vi "Custom Aggregation (Symm Comp).vi"(0 "symmetrical components":T2, 1 "reset? (F)":bool, 5 "aggregation settings":T1={"interval"=1, "interval unit"=enum."Runs", "synchronization of intervals"=enum."Not synchronized", "algorithm"=enum."Average"}, 9 "system info in":refnum<class "EP System Info.lvclass">, 11 "error in (no error)":errorcluster, 12 "data timestamp":timestamp) -> (4 "aggregated minimum value":T2, 6 "aggregated averaged/RMS value":T2, 8 "aggregated maximum value":T2, 10 "system info out":refnum<class "EP System Info.lvclass">, 13 "aggregated data valid?":bool, 14 "aggregated data timestamp":timestamp, 15 "error out":errorcluster)   [LabVIEW 2014, in "NI_EP_Power Quality.lvlib"]
doc: "Calculates the aggregated minimum, maximum, and averaged or RMS value of an input signal for a specified aggregation interval, according to Class S in IEC 61000-4-30:2008. There is no overlap between aggregation intervals. This VI automatically restarts accumulation at the beginning of the next time interval after the previous interval expires. You must manually select the polymorphic instance you want to use.\n\nThis VI supports measuring single-line and multiple-line systems except the DBL instance. Use the DBL instance to measure one channel on one line at one time."
uses:
  <vilib>/addons/Electrical Power/PQ/NI_EP_Power Quality.lvlib
  <vilib>/addons/Electrical Power/PQ/Common/Controls/ep_Aggregation Settings.ctl
  <vilib>/addons/Electrical Power/PQ/Common/Classes/System Info/EP System Info.lvclass
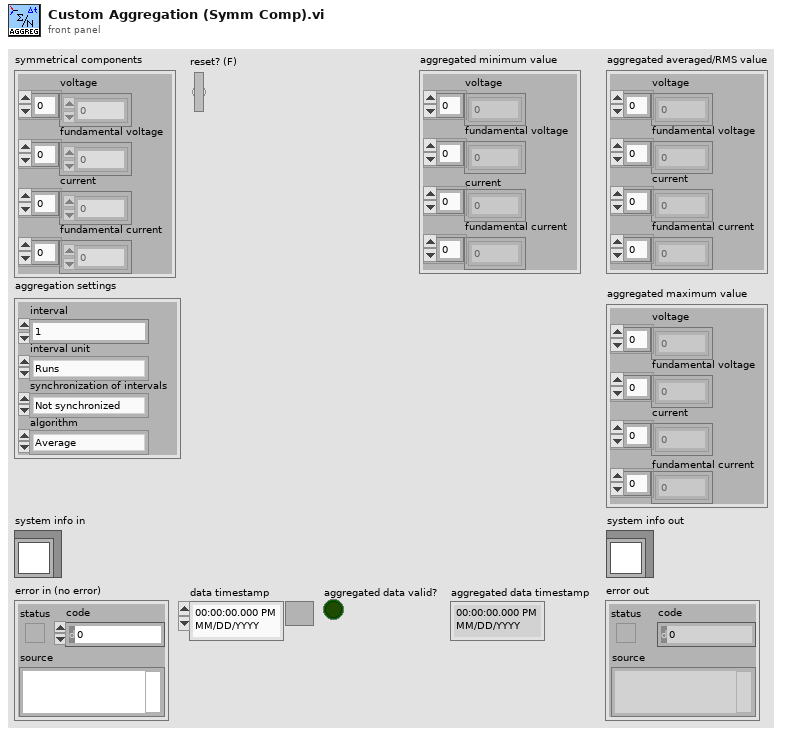
[diagram p1: front panel]
types:
  T1 = typedef "NI_EP_Power Quality.lvlib/ep_Aggregation Settings.ctl" = cluster{"interval":u32, "interval unit":enum16{"Runs", "Seconds", "Minutes", "Hours", "Days", "Weeks"}, "synchronization of intervals":enum16{"Not synchronized", "Interval rounded"}, "algorithm":enum16{"Average", "RMS"}}
  T2 = cluster{"voltage":dbl[], "fundamental voltage":dbl[], "current":dbl[], "fundamental current":dbl[]}
  T3 = cluster{"aggregated minimum values":dbl[], "aggregated minimum values":dbl[], "aggregated minimum values":dbl[], "aggregated minimum values":dbl[]}
  T4 = cluster{"aggregated averaged/RMS values":dbl[], "aggregated averaged/RMS values":dbl[], "aggregated averaged/RMS values":dbl[], "aggregated averaged/RMS values":dbl[]}
  T5 = cluster{"aggregated maximum values":dbl[], "aggregated maximum values":dbl[], "aggregated maximum values":dbl[], "aggregated maximum values":dbl[]}
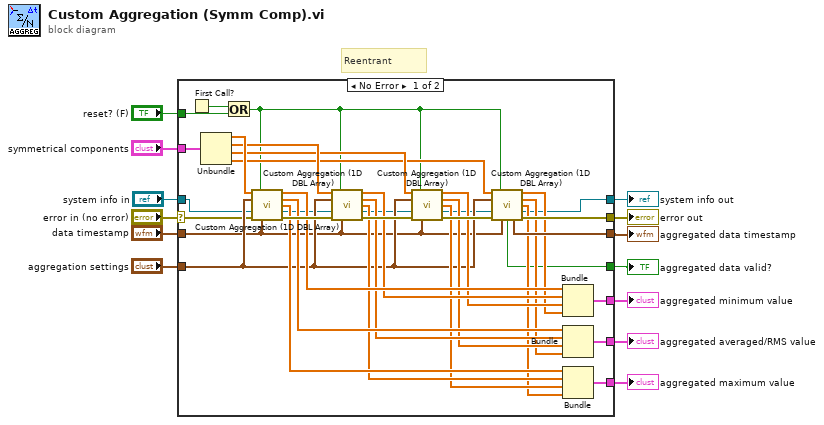
[diagram p0: block diagram]
diagram:
  # "Reentrant"
  n1 = case shown="No Error" "error in (no error)" {
    selector: "error in (no error)" -> [w23 w52]
    tunnel: "reset? (F)" -> [w21 _]
    tunnel: [w47 w52] -> w12
    tunnel: [w46 _] -> w4
    tunnel: "symmetrical components" -> [w45 _]
    tunnel: [w44 _] -> w10
    tunnel: [w43 _] -> w9
    tunnel: [w42 _] -> w8
    tunnel: "data timestamp" -> [w19 _]
    tunnel: "aggregation settings" -> [w28 _]
    tunnel: [w24 _] -> w3
    tunnel: "system info in" -> [w18 w51]
    tunnel: [w14 w51] -> w1
    frame No Error {
      n2 = First Call?() -> (First Call?: T/F=w22:bool)
      n3 = Unbundle(w45) -> ("voltage"=w41:dbl[], "fundamental voltage"=w37:dbl[], "current"=w33:dbl[], "fundamental current"=w29:dbl[])
      n4 = Or(x=w22, y=w21) -> (x .or. y?=w20:bool)
      n5 = call <vilib>:"Custom Aggregation (1D DBL Array).vi"("data in"=w41, "reset? (F)"=w20, "aggregation settings"=w28, "system info in"=w18, "error in (no error)"=w23, "data timestamp"=w19) -> ("aggregated minimum values"=w40:dbl[], "aggregated averaged/RMS values"=w39:dbl[], "aggregated maximum values"=w38:dbl[], "system info out"=w17:refnum<class "EP System Info.lvclass">, "error out"=w50:errorcluster)  [unwired: 3 in, 2 out]
      n6 = call <vilib>:"Custom Aggregation (1D DBL Array).vi"("data in"=w37, "reset? (F)"=w20, "aggregation settings"=w28, "system info in"=w17, "error in (no error)"=w50, "data timestamp"=w19) -> ("aggregated minimum values"=w36:dbl[], "aggregated averaged/RMS values"=w35:dbl[], "aggregated maximum values"=w34:dbl[], "system info out"=w16:refnum<class "EP System Info.lvclass">, "error out"=w49:errorcluster)  [unwired: 3 in, 2 out]
      n7 = call <vilib>:"Custom Aggregation (1D DBL Array).vi"("data in"=w33, "reset? (F)"=w20, "aggregation settings"=w28, "system info in"=w16, "error in (no error)"=w49, "data timestamp"=w19) -> ("aggregated minimum values"=w32:dbl[], "aggregated averaged/RMS values"=w31:dbl[], "aggregated maximum values"=w30:dbl[], "system info out"=w15:refnum<class "EP System Info.lvclass">, "error out"=w48:errorcluster)  [unwired: 3 in, 2 out]
      n8 = call <vilib>:"Custom Aggregation (1D DBL Array).vi"("data in"=w29, "reset? (F)"=w20, "aggregation settings"=w28, "system info in"=w15, "error in (no error)"=w48, "data timestamp"=w19) -> ("aggregated minimum values"=w27:dbl[], "aggregated averaged/RMS values"=w26:dbl[], "aggregated maximum values"=w25:dbl[], "system info out"=w14:refnum<class "EP System Info.lvclass">, "aggregated data valid?"=w24:bool, "aggregated data timestamp"=w46:timestamp, "error out"=w47:errorcluster)  [unwired: 3 in]
      n9 = Bundle("aggregated minimum values"=w40, "aggregated minimum values"=w36, "aggregated minimum values"=w32, "aggregated minimum values"=w27) -> (w44:T3)  [unwired: 1 in]
      n10 = Bundle("aggregated averaged/RMS values"=w39, "aggregated averaged/RMS values"=w35, "aggregated averaged/RMS values"=w31, "aggregated averaged/RMS values"=w26) -> (w43:T4)  [unwired: 1 in]
      n11 = Bundle("aggregated maximum values"=w38, "aggregated maximum values"=w34, "aggregated maximum values"=w30, "aggregated maximum values"=w25) -> (w42:T5)  [unwired: 1 in]
    }
    frame Error {
    }
  }
  "aggregated minimum value" <- w10
  "aggregated averaged/RMS value" <- w9
  "aggregated maximum value" <- w8
  "error out" <- w12
  "aggregated data valid?" <- w3
  "aggregated data timestamp" <- w4
  "system info out" <- w1
